vi "soundB.vi"(8 "check":bool, 9 "Ack2":bool, 10 "Ack1":bool, 11 "alr":bool[](array[boolean])) -> (3 "sound":bool)   [LabVIEW 2019, in "Alarms.lvlib"]
uses:
  Alarms.lvlib
  Trigers/Triggers.lvlib
  Logik/Logik.lvlib
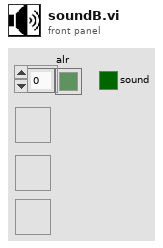
[diagram p1: front panel]
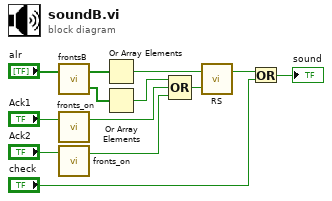
[diagram p0: block diagram]
diagram:
  n1 = call "frontsB.vi"("IN"="alr") -> ("FALL"=w2:bool[], "RAISE"=w7:bool[])  [unwired: 1 in]
  n2 = call "fronts_on.vi"("in"="Ack1") -> ("raise"=w5:bool)  [unwired: 1 in, 1 out]
  n3 = call "fronts_on.vi"("in"="Ack2") -> ("raise"=w3:bool)  [unwired: 1 in, 1 out]
  n4 = Or Array Elements(Boolean array=w7) -> (logical OR=w9:bool)
  n5 = Or Array Elements(Boolean array=w2) -> (logical OR=w1:bool)
  n6 = Compound Arithmetic op=OR(w1, w5, w3) -> (w13:bool)
  n7 = call "RS.vi"("R"=w13, "S"=w9) -> ("Q"=w12:bool)  [unwired: 1 out]
  n8 = Or(x=w12, y="check") -> (x .or. y?=→"sound":bool)
